vi "Init.vi"(8 "error in (no error)":errorcluster, 9 "Config File Path":path=path "", 10 "Name":string, 11 "Test Runner In":refnum<class "Test Runner.lvclass">) -> (0 "error out":errorcluster, 3 "Test Runner Out":refnum<class "Test Runner.lvclass">)   [LabVIEW 2020, in "Test Runner.lvclass"]
uses:
  Test Runner.lvclass
  Application Framework/Process Classes/Process/Process.lvclass
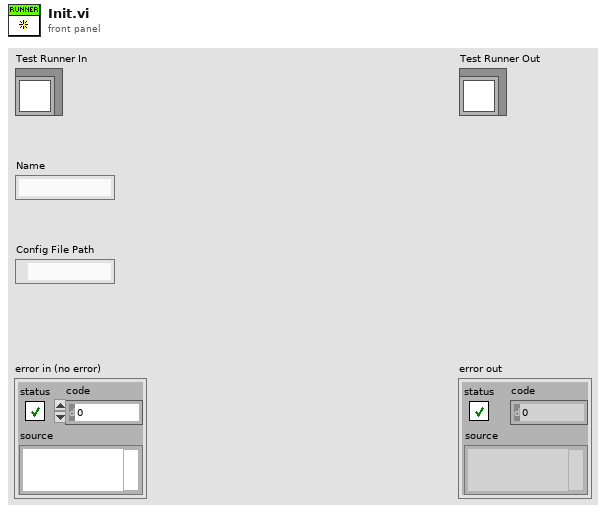
[diagram p1: front panel]
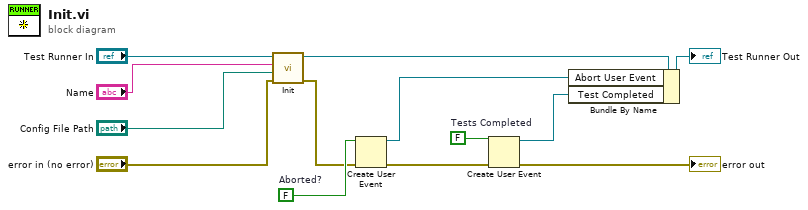
[diagram p0: block diagram]
diagram:
  w3 = FALSE  # Tests Completed
  w9 = FALSE  # Aborted?
  n1 = call-parent "Init.vi"("error in (no error)"="error in (no error)", "Config File Path"="Config File Path", "Name"="Name", "Process In"="Test Runner In") -> ("error out"=w7:errorcluster, "Process Out"=w12:refnum<class "Test Runner.lvclass">)  [unwired: 6 in]
  n2 = Create User Event(user event datatype=w9, error in=w7) -> (user event=w8:refnum<user-event>, error out=w6:errorcluster)
  n3 = Create User Event(user event datatype=w3, error in=w6) -> (user event=w1:refnum<user-event>, error out=→"error out":errorcluster)
  n4 = Bundle By Name(cluster=w12, "Abort User Event"=w8, "Test Completed"=w1) -> (→"Test Runner Out":refnum<class "Test Runner.lvclass">)
